vi "06 Panels in panels.vi"() -> ()   [LabVIEW 2019]
uses:
  _Subs/OpenDiagram/Open_XControl.xctl
panel:
  in  "Stop Button":bool
  in  "OpenDiag":refnum<vi>(xcontrol)
  # "06 Panels within Panels\nThis code lets you run a program within another\n\nInstructions:\n1. Hit the Run arrow and see the Gauge change to the value of the Slide\n2. Hit Continuous Run and watch the Gauge change as you vary the Slide"
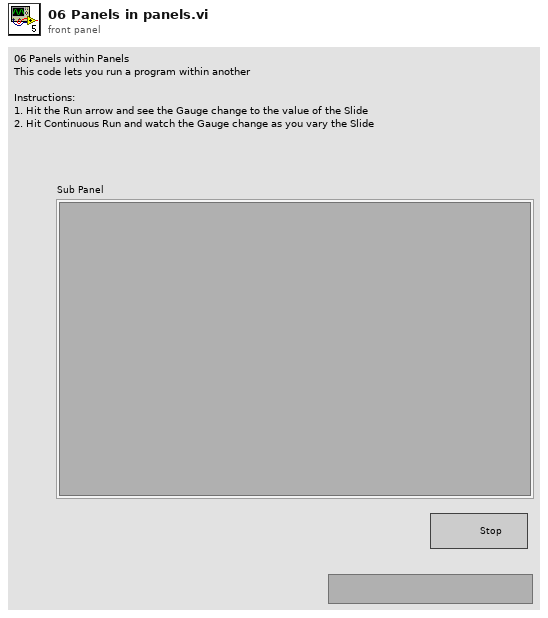
[diagram p1: front panel]
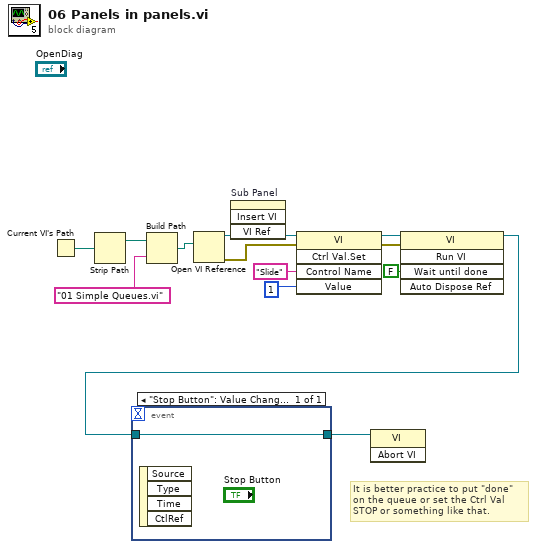
[diagram p0: block diagram]
diagram:
  # "It is better practice to put \"done\"\non the queue or set the Ctrl Val\nSTOP or something like that."
  n1 = Current VI's Path() -> (path=w13:path)
  n2 = Strip Path(path=w13) -> (stripped path=w10:path)  [unwired: 1 out]
  n3 = Build Path(base path=w10, name or relative path="01 Simple Queues.vi") -> (appended path=w12:path)
  n4 = Open VI Reference(vi path=w12) -> (vi reference=w2:refnum<vi>, error out=w11:errorcluster)  [unwired: 5 in]
  n5 = invoke on="Sub Panel" class="SubPnl" method="Insert VI"("VI Ref"=w2) -> ()  [unwired: 3 in, 4 out]
  n6 = invoke class="VI" method="Ctrl Val.Set"(reference=w2, error in=w11, "Control Name"="Slide", "Value"=1) -> (reference out=w6:refnum<vi>, error out=w5:errorcluster)  [unwired: 1 in, 3 out]
  n7 = invoke class="VI" method="Run VI"(reference=w6, error in=w5, "Wait until done"=FALSE ("Wait Until Done")) -> (reference out=w3:refnum<vi>)  [unwired: 2 in, 4 out]
  n8 = event shown="[0] \"Stop Button\": Value Change" {
    selector: _ -> [_]
    dyn-events: _ -> [_]
    timeout: _ -> [_]
    tunnel: [w14] -> w4
    tunnel: w3 -> [w14]
    event "Stop Button": Value Change {
      n9 = event-data() -> ()  [unwired: 1 in, 4 out]
    }
  }
  n10 = invoke class="VI" method="Abort VI"(reference=w4) -> ()  [unwired: 2 in, 3 out]
